vi "ChangeHeadDir.vi"(8 "error in (no error)":errorcluster, 10 "UnitDirection":T1, 11 "SnakeBodyCell in":refnum<class "SnakeBodyCell.lvclass">) -> (0 "error out":errorcluster, 3 "SnakeBodyCell out":refnum<class "SnakeBodyCell.lvclass">)   [LabVIEW 2018, in "SnakeBodyCell.lvclass"]
uses:
  SnakeBodyCell.lvclass
  Typedefs/UnitDirection.ctl
  SnakeBodyCell.lvclass/SnakeBodyCell.ctl
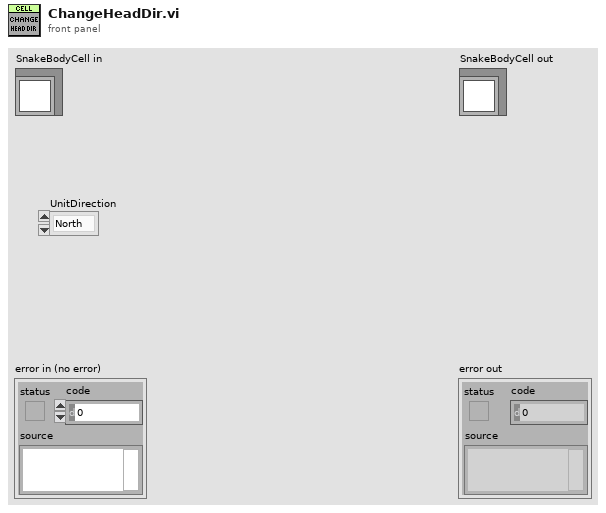
[diagram p1: front panel]
types:
  T1 = typedef "UnitDirection.ctl" = enum16{"North", "East", "South", "West"}
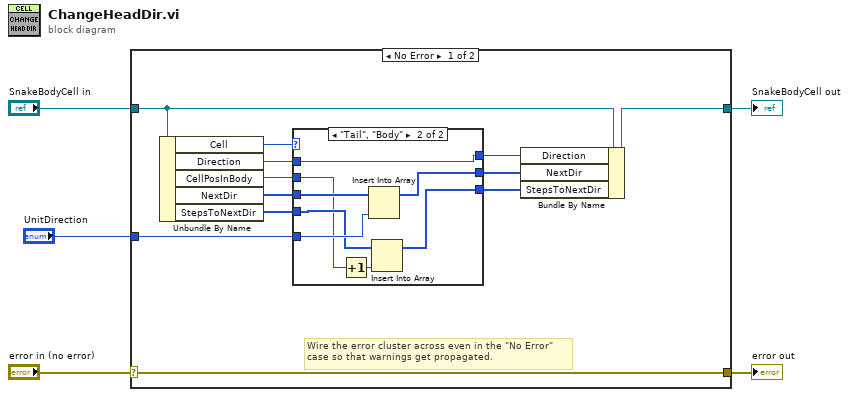
[diagram p0: block diagram]
diagram:
  n1 = case shown="No Error" "error in (no error)" {
    selector: "error in (no error)" -> [w17 w30]
    tunnel: [w17 w30] -> w4
    tunnel: [w15 w29] -> w2
    tunnel: "SnakeBodyCell in" -> [w16 w29]
    tunnel: "UnitDirection" -> [w13 _]
    frame No Error {
      # "Wire the error cluster across even in the \"No Error\"\ncase so that warnings get propagated."
      n2 = Unbundle By Name(w16) -> ("Cell"=w14:enum16{"Head", "Tail", "Body"}, "Direction"=w6:T1, "CellPosInBody"=w11:u16, "NextDir"=w10:T1[], "StepsToNextDir"=w9:u16[])
      n3 = case shown="\"Tail\", \"Body\"" w14 {
        tunnel: w13 -> [w20 w27]
        tunnel: [w20 w22] -> w12
        tunnel: w11 -> [_ w24]
        tunnel: w10 -> [w19 w28]
        tunnel: w9 -> [w18 w26]
        tunnel: [w18 w25] -> w8
        tunnel: [w19 w23] -> w7
        tunnel: w6 -> [_ w22]
        frame "Head", Default {
        }
        frame "Tail", "Body" {
          n4 = Increment(x=w24) -> (x+1=w21:u16)
          n5 = Insert Into Array(array=w28, new element=w27) -> (w23:T1[])  [unwired: 1 in]
          n6 = Insert Into Array(array=w26, new element=w21) -> (w25:u16[])  [unwired: 1 in]
        }
      }
      n7 = Bundle By Name(cluster=w16, "Direction"=w12, "NextDir"=w7, "StepsToNextDir"=w8) -> (w15:refnum<class "SnakeBodyCell.lvclass">)
    }
    frame Error {
    }
  }
  "error out" <- w4
  "SnakeBodyCell out" <- w2
